vi "Write JSON Config.vi"(6 "Pretty Print?":bool, 8 "error in (no error)":errorcluster, 11 "AbsFunc_Two Term_U32 in":refnum<class "AbsFunc_Two Term_U32.lvclass">) -> (0 "error out":errorcluster, 2 "JSON":string, 3 "AbsFunc_Two Term_U32 out":refnum<class "AbsFunc_Two Term_U32.lvclass">)   [LabVIEW 2021, in "AbsFunc_Two Term_U32.lvclass"]
uses:
  AbsFunc_Two Term_U32.lvclass
  C:/Program Files (x86)/National Instruments/LabVIEW 2021/vi.lib/TSA/Abstract Data Classes/Abs_Types/Type/Abs_Type.lvclass
  AbsFunc_Two Term_U32.lvclass/AbsFunc_Two Term_U32.ctl
  <vilib>/JDP Science/JSONtext/Make JSON Array.vi
  <vilib>/JDP Science/JSONtext/Merge into Object.vi
  <vilib>/JDP Science/JSONtext/Make JSON Object.vi
  <vilib>/Utility/LVClass/Get LV Class Name.vi
  <vilib>/JDP Science/JSONtext/support/Format JSON Array Text.vi
  <vilib>/JDP Science/JSONtext/support/Format JSON Object.vi
  <vilib>/JDP Science/JSONtext/Get all Object Items.vi
  <vilib>/JDP Science/JSONtext/Set Multiple Object Items.vi
  Abs_Types/U32 Integer/Abs_U32 Integer.lvclass
  Abs_Types/Numeric/Abs_Numeric.lvclass
  Abs_Types/Type/Abs_Type.lvclass
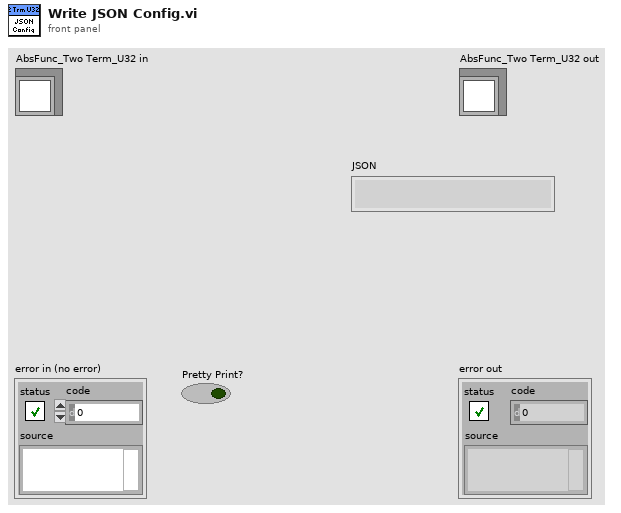
[diagram p1: front panel]
types:
  T1 = typedef "AbsFunc_Two Term_U32.lvclass/Abstract Type.ctl" = refnum<class "Abs_U32 Integer.lvclass">
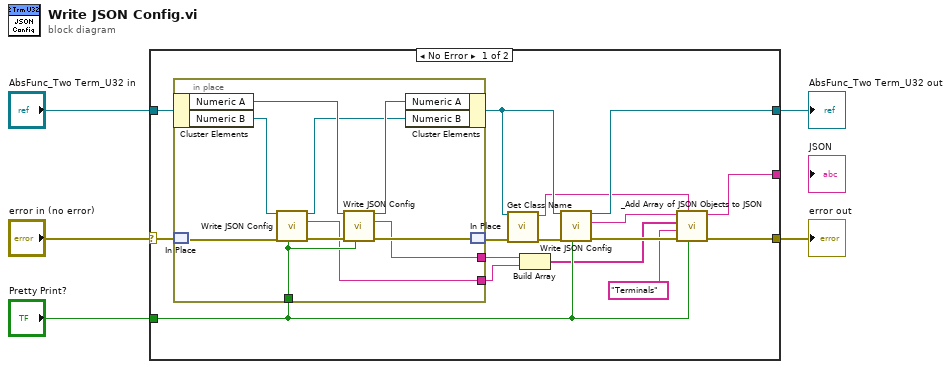
[diagram p0: block diagram]
diagram:
  n1 = case shown="No Error" "error in (no error)" {
    selector: "error in (no error)" -> [w16 w33]
    tunnel: "AbsFunc_Two Term_U32 in" -> [w21 w32]
    tunnel: [w20 w32] -> w1
    tunnel: [w12 _] -> _
    tunnel: [w11 w33] -> w2
    tunnel: "Pretty Print?" -> [w10 _]
    frame No Error {
      n2 = in-place {
        in-place-border: w10 -> [w29]
        in-place-border: [w27] -> w19
        in-place-border: [w26] -> w18
        n3 = in-place-cluster #1(w21) -> ("Numeric A"=w25:T1, "Numeric B"=w23:refnum<class "Abs_Numeric.lvclass">)
        n4 = in-place-match #2(w16) -> (w30:errorcluster)
        n5 = call-dynamic "Write JSON Config.vi"("Pretty Print?"=w29, "error in (no error)"=w30, "Abs_Type in"=w23) -> ("error out"=w31:errorcluster, "JSON"=w26:string, "Abs_Type out"=w22:refnum<class "Abs_Numeric.lvclass">)  [unwired: 6 in]
        n6 = call-dynamic "Write JSON Config.vi"("Pretty Print?"=w29, "error in (no error)"=w31, "Abs_Type in"=w25) -> ("error out"=w28:errorcluster, "JSON"=w27:string, "Abs_Type out"=w24:T1)  [unwired: 6 in]
        n7 = in-place-cluster #1("Numeric A"=w24, "Numeric B"=w22) -> (w14:refnum<class "AbsFunc_Two Term_U32.lvclass">)
        n8 = in-place-match #2(w28) -> (w17:errorcluster)
      }
      n9 = call "Get Class Name.vi"("error in (no error)"=w17, "Abs_Type in"=w14) -> ("error out"=w15:errorcluster, "class name"=w9:string)  [unwired: 8 in]
      n10 = Build Array(w19, w18) -> (w7:string[])
      n11 = call-parent "Write JSON Config.vi"("Pretty Print?"=w10, "error in (no error)"=w15, "Abs_Type in"=w14) -> ("error out"=w13:errorcluster, "JSON"=w8:string, "Abs_Type out"=w20:refnum<class "AbsFunc_Two Term_U32.lvclass">)  [unwired: 6 in]
      n12 = call "_Add Array of JSON Objects to JSON.vi"("Pretty Print?"=w10, "JSON Object Name"=w9, "error in (no error)"=w13, "JSON Array Name"="Terminals", "JSON Objects"=w7, "JSON"=w8) -> ("error out"=w11:errorcluster, "<JSON>"=w12:string)  [unwired: 4 in]
    }
    frame Error {
    }
  }
  "error out" <- w2
  "AbsFunc_Two Term_U32 out" <- w1
